vi "Set Power.vi"(8 "error in (no error)":errorcluster, 10 "Power":dbl, 11 "Laser Controller API in":refnum<class "Laser Controller.lvclass">) -> (0 "error out":errorcluster, 3 "Laser Controller API out":refnum<class "Laser Controller.lvclass">)   [LabVIEW 2022 SP3, in "Laser Controller.lvclass"]
uses:
  Laser Controller.lvclass
  Laser Controller.lvclass/Laser Controller.ctl
  Laser State Data/Laser State Data.lvclass/Laser State Data.ctl
  Laser Process/Laser Process Messages/Set Power Msg/Set Power Msg.lvclass/Set Power Msg.ctl
  Laser State Data/Read Laser State.vi
  Laser Process/Laser Process Messages/Set Power Msg/Set Power Msg.lvclass
  C:/Program Files/National Instruments/LabVIEW 2022/vi.lib/ActorFramework/Message/Message.lvclass
  <vilib>/Utility/error.llb/Error Cluster From Error Code.vi
  <vilib>/ErrorRing/Error Ring.xnode
  XY Stage/Process Actor/Process Framework/Interlock Q Class/Interlock Q Class.lvclass
  Laser State Data/Laser State Data.lvclass
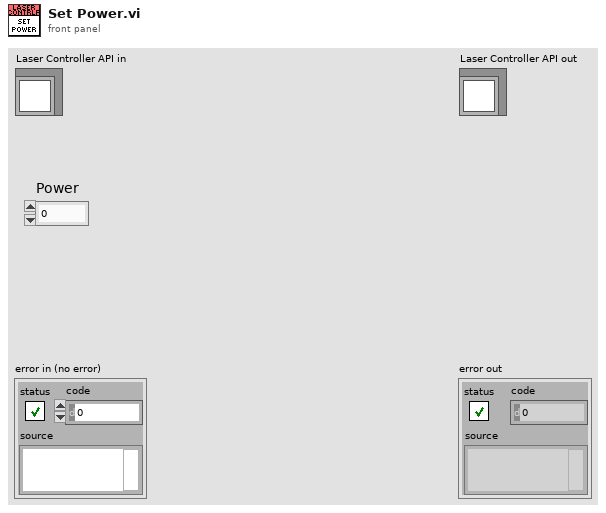
[diagram p1: front panel]
types:
  T1 = typedef "Laser State Data.lvclass/Laser State.ctl" = enum16{"Idle", "Warming", "Ready", "Firing"}
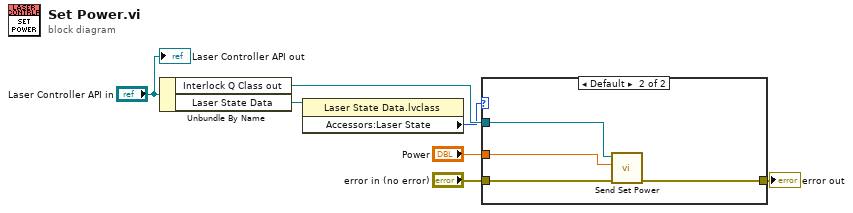
[diagram p0: block diagram]
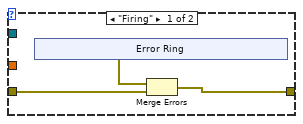
[diagram p2: hidden frame]
diagram:
  n1 = Unbundle By Name("Laser Controller API in") -> ("Interlock Q Class out"=w6:refnum<class "Interlock Q Class.lvclass">, "Laser State Data"=w2:refnum<data-value>)
  n2 = property class="Laser State Data.lvclass"(reference=w2) -> ("Accessors:Laser State"=w1:T1)  [unwired: 1 in, 2 out]
  n3 = case shown="Default" w1 {
    tunnel: w6 -> [_ w19]
    tunnel: "Power" -> [_ w18]
    tunnel: "error in (no error)" -> [w10 w17]
    tunnel: [w9 w16] -> w3
    frame "Firing" {
      n4 = xnode "Error Ring"() -> ("error out"=w8:errorcluster)
      n5 = Merge Errors(w8, w10) -> (w9:errorcluster)
    }
    frame Default {
      n6 = call "Send Set Power.vi"("error in (no error)"=w17, "Power"=w18, "Interlock Q Class in"=w19) -> ("error out"=w16:errorcluster)  [unwired: 7 in, 1 out]
    }
  }
  "error out" <- w3
  "Laser Controller API out" <- "Laser Controller API in"
